vi "GetCurrentLocalization.vi"() -> (0 "Current Localization Status":T2={"x"=3.3217286864690756, "y"=1.792930753359125, "angle"=4.188260232231081, "valid"=TRUE, "lastUpdatedTime"=370860344.0}, 1 "Current Localization Vector":T1={"x"=3.3217286864690756, "y"=1.792930753359125, "angle"=4.188260232231081})   [LabVIEW 2015]
doc: "Gets current localization info from Shared Variable Engine. This SHOULD BE the only VI you have to change if you change how the Localization System communicates over the SVE."
uses:
  LocalizationStatus.ctl
  Vector.ctl
  Navigation2017.lvlib
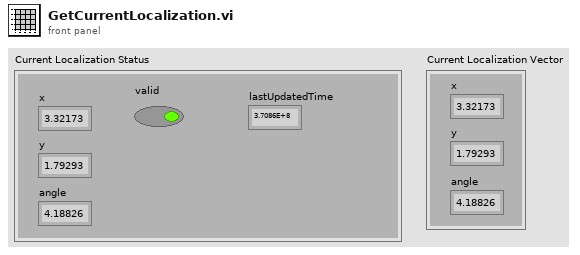
[diagram p1: front panel]
types:
  T1 = typedef "Navigation2017.lvlib/Vector.ctl" = cluster{"x":dbl, "y":dbl, "angle":dbl}
  T2 = typedef "LocalizationStatus.ctl" = cluster{"x":dbl, "y":dbl, "angle":dbl, "valid":bool, "lastUpdatedTime":dbl}
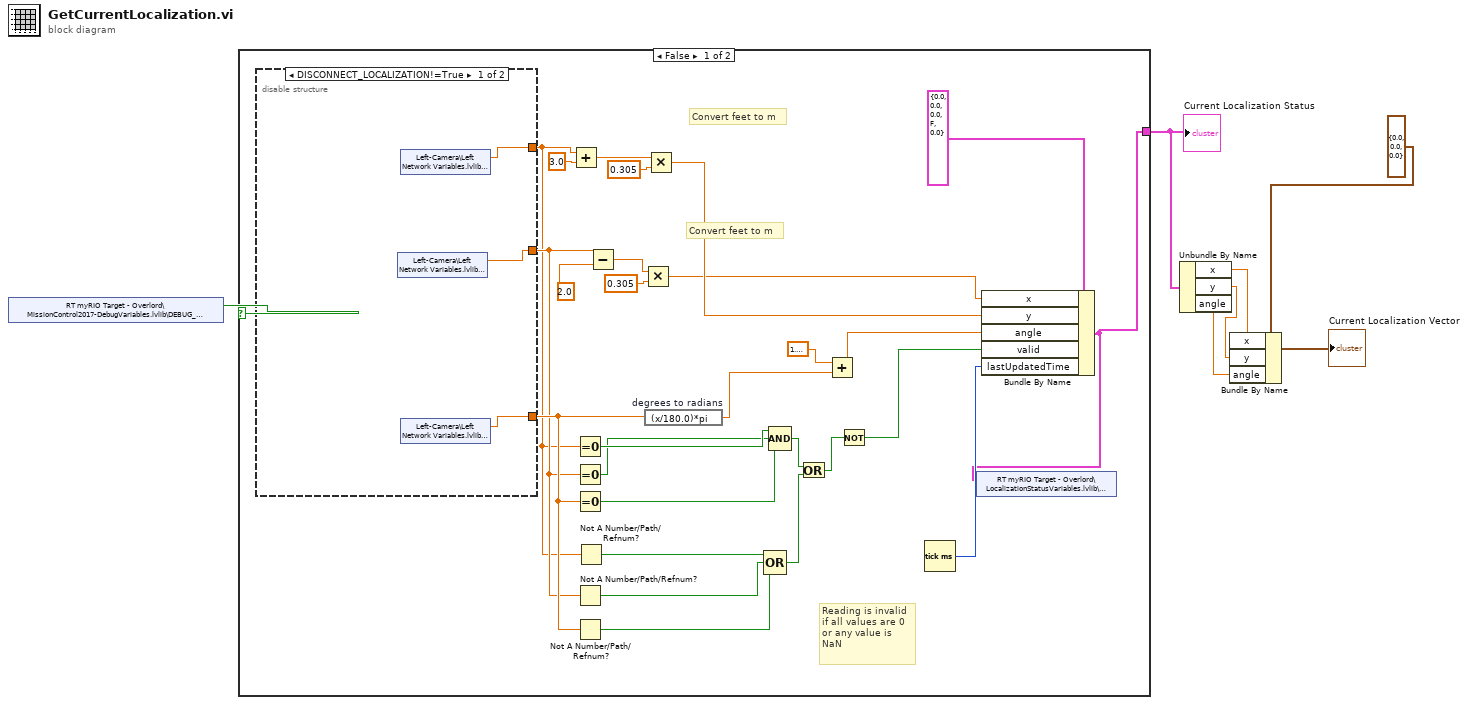
[diagram p0: block diagram]
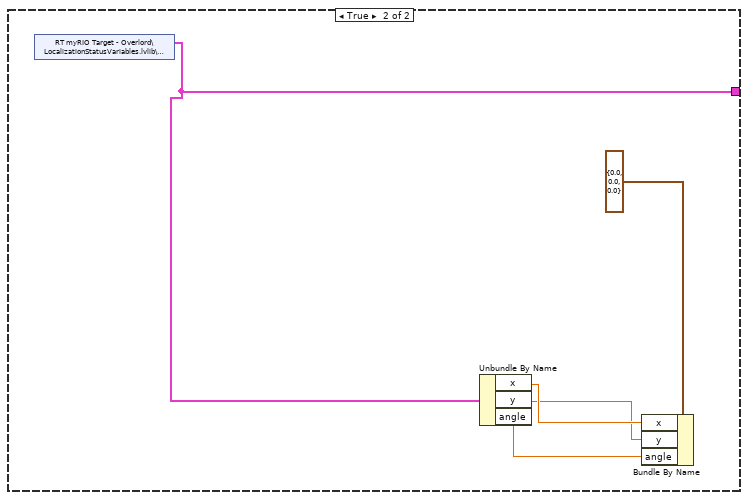
[diagram p3: hidden frame]
diagram:
  n1 = shared-variable "RT myRIO Target - Overlord\\MissionControl2017-DebugVariables.lvlib\\DEBUG_LOCALIZATION_MOUSE"() -> (w1:bool)  [unwired: 1 in, 1 out]
  n2 = case shown="False" w1 {
    tunnel: [w31 w38] -> w7
    frame False {
      # "Reading is invalid\nif all values are 0\nor any value is \nNaN"
      # "Convert feet to m"
      # "Convert feet to m"
      n3 = disable-structure shown="DISCONNECT_LOCALIZATION!=True" {
        disable-tunnel: [w37 _] -> w9
        disable-tunnel: [w35 _] -> w11
        disable-tunnel: [w36 _] -> w10
        frame condition #0 (active) {
          n4 = shared-variable "Left-Camera\\Left Network Variables.lvlib\\Center Y"() -> (w36:dbl)  [unwired: 1 in, 1 out]
          n5 = shared-variable "Left-Camera\\Left Network Variables.lvlib\\Center X"() -> (w37:dbl)  [unwired: 1 in, 1 out]
          n6 = shared-variable "Left-Camera\\Left Network Variables.lvlib\\Heading"() -> (w35:dbl)  [unwired: 1 in, 1 out]
        }
        frame condition #1 {
        }
      }
      n7 = Add(x=w9, y=3.0) -> (x+y=w28:dbl)
      n8 = Equal To 0?(x=w9) -> (x = 0?=w19:bool)
      n9 = Equal To 0?(x=w10) -> (x = 0?=w18:bool)
      n10 = Equal To 0?(x=w11) -> (x = 0?=w17:bool)
      n11 = Not A Number/Path/Refnum?(number/path/refnum=w10) -> (NaN/Path/Refnum?=w13:bool)
      n12 = Not A Number/Path/Refnum?(number/path/refnum=w11) -> (NaN/Path/Refnum?=w12:bool)
      n13 = Not A Number/Path/Refnum?(number/path/refnum=w9) -> (NaN/Path/Refnum?=w14:bool)
      n14 = Subtract(x=w10, y=2.0) -> (x-y=w25:dbl)
      n15 = Multiply(x=w25, y=0.305) -> (x*y=w26:dbl)
      n16 = expression code="(x/180.0)*pi" "degrees to radians"(w11) -> (w23:dbl)
      n17 = Multiply(x=w28, y=0.305) -> (x*y=w29:dbl)
      n18 = Compound Arithmetic op=OR(w14, w13, w12) -> (w8:bool)
      n19 = Compound Arithmetic op=AND(w19, w18, w17) -> (w16:bool)
      n20 = Or(x=w16, y=w8) -> (x .or. y?=w15:bool)
      n21 = Add(x=1.5707963267948966, y=w23) -> (x+y=w22:dbl)
      n22 = Not(x=w15) -> (.not. x?=w20:bool)
      n23 = Tick Count (ms)() -> (millisecond timer value=w32:u32)
      n24 = Bundle By Name(cluster=T2 {"x"=0.0, "y"=0.0, "angle"=0.0, "valid"=FALSE, "lastUpdatedTime"=0.0} ("Localization Status"), "x"=w26, "y"=w29, "angle"=w22, "valid"=w20, "lastUpdatedTime"=w32) -> (w31:T2)
      n25 = shared-variable "RT myRIO Target - Overlord\\LocalizationStatusVariables.lvlib\\LocalizationStatus"(w31) -> ()  [unwired: 1 in, 1 out]
    }
    frame True {
      n26 = shared-variable "RT myRIO Target - Overlord\\LocalizationStatusVariables.lvlib\\LocalizationStatus"() -> (w38:T2)  [unwired: 1 in, 1 out]
      n27 = Unbundle By Name(w38) -> ("x"=w41:dbl, "y"=w40:dbl, "angle"=w39:dbl)
      n28 = Bundle By Name(cluster=T1 {"x"=0.0, "y"=0.0, "angle"=0.0} ("Vector"), "x"=w41, "y"=w40, "angle"=w39) -> ()  [unwired: 1 out]
    }
  }
  "Current Localization Status" <- w7
  n29 = Unbundle By Name(w7) -> ("x"=w4:dbl, "y"=w3:dbl, "angle"=w2:dbl)
  n30 = Bundle By Name(cluster=T1 {"x"=0.0, "y"=0.0, "angle"=0.0} ("Vector"), "x"=w4, "y"=w3, "angle"=w2) -> (→"Current Localization Vector":T1)
